vi "ReadStatus.vi"(0 "object in":refnum<class "CetoniPump.lvclass">, 5 "error in (no error)":errorcluster) -> (14 "object out":refnum<class "CetoniPump.lvclass">, 16 "Fill Level":dbl, 17 "Is pumping":bool, 18 "Actual Flow Rate":dbl, 19 "error out":errorcluster)   [LabVIEW 2021, in "CetoniPump.lvclass"]
uses:
  CetoniPump.lvclass
  CetoniPump.lvclass/CetoniPump.ctl
  Users/olaja/AppData/Local/CETONI_SDK/lib/labview/labbCAN_Pump_API/labbCAN_Pump_API.lvlib
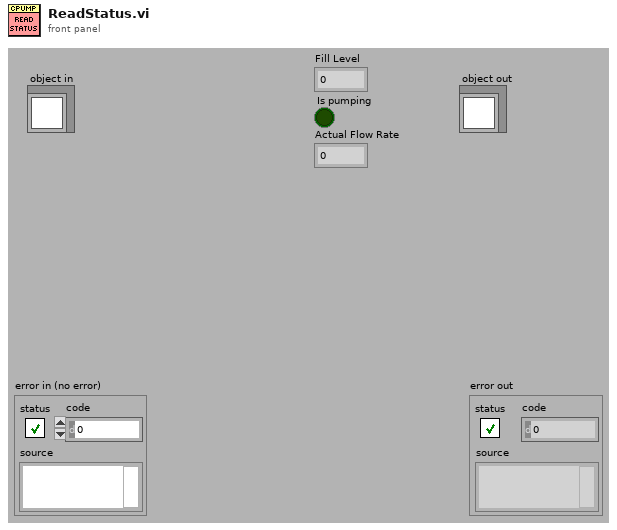
[diagram p1: front panel]
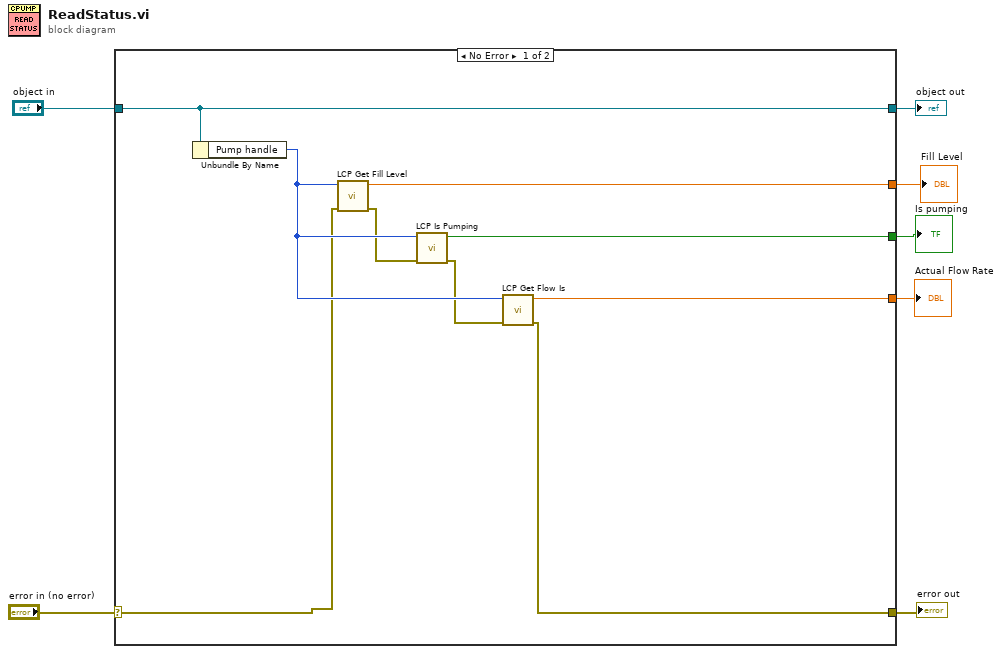
[diagram p0: block diagram]
diagram:
  n1 = case shown="No Error" "error in (no error)" {
    selector: "error in (no error)" -> [w10 w18]
    tunnel: [w9 w18] -> w6
    tunnel: [w16 w17] -> w4
    tunnel: "object in" -> [w16 w17]
    tunnel: [w15 _] -> w3
    tunnel: [w14 _] -> w2
    tunnel: [w8 _] -> w1
    frame No Error {
      n2 = Unbundle By Name(w16) -> ("Pump handle"=w13:i64)
      n3 = call "LCP Get Fill Level.vi"("error in (no error)"=w10, "Pump Handle"=w13) -> ("error out"=w12:errorcluster, "Fill Level"=w15:dbl)  [unwired: 8 in]
      n4 = call "LCP Is Pumping.vi"("error in (no error)"=w12, "Pump Handle"=w13) -> ("error out"=w11:errorcluster, "Is pumping"=w14:bool)  [unwired: 8 in]
      n5 = call "LCP Get Flow Is.vi"("error in (no error)"=w11, "Pump Handle"=w13) -> ("error out"=w9:errorcluster, "Actual Flow Rate"=w8:dbl)  [unwired: 8 in]
    }
    frame Error {
    }
  }
  "error out" <- w6
  "object out" <- w4
  "Fill Level" <- w3
  "Is pumping" <- w2
  "Actual Flow Rate" <- w1
